vi "programacion 4 tercer parcial.vi"() -> ()   [LabVIEW 2011]
panel:
  out "Array":dbl[](array[numeric])
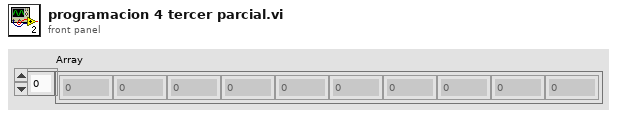
[diagram p1: front panel]
types:
  T1 = enum16{"open", "replace", "create", "open or create", "replace or create", "replace or create with confirmation"}
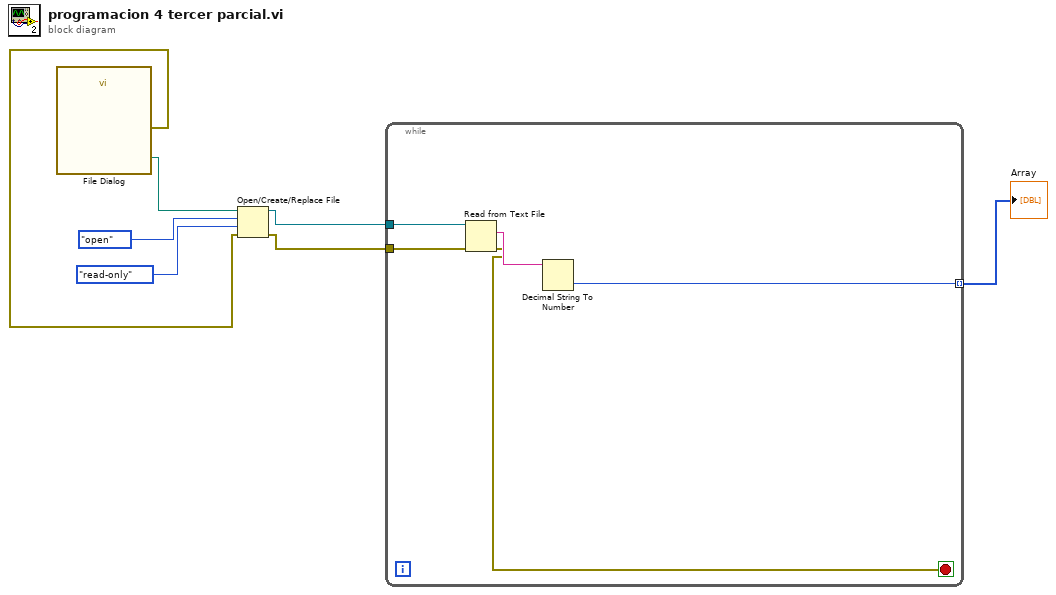
[diagram p0: block diagram]
diagram:
  n1 = call "File Dialog"() -> ("selected path"=w7:path, "error out"=w4:errorcluster)  [unwired: 12 in, 2 out]
  n2 = Open/Create/Replace File(file path (use dialog)=w7, error in=w4, operation (0:open)=T1."open", access (0:read/write)=enum16{"read/write", "read-only", "write-only"}."read-only") -> (refnum out=w2:refnum<file>, error out=w3:errorcluster)  [unwired: 2 in, 1 out]
  n3 = while {
    tunnel: w3 -> [w12]
    tunnel: w2 -> [w11]
    tunnel: [w9] -> w1 mode=indexing
    stop <- w8 stop-if-true
    n4 = Read from Text File(file (use dialog)=w11, error in=w12) -> (text=w10:string, error out=w8:errorcluster)  [unwired: 2 in, 2 out]
    n5 = Decimal String To Number(string=w10) -> (number=w9:i32)  [unwired: 2 in, 1 out]
  }
  "Array" <- w1
